vi "Plotsettings.vi"(4 "Decays 2":refnum<vi>, 5 "No of Channels":u32) -> ()   [LabVIEW 2009]
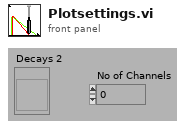
[diagram p1: front panel]
types:
  T1 = typedef "Settings.ctl" = cluster{"threshold":cluster{"max":u32, "min":u32}, "RGB or false color":bool, "16bit":bool, "log/lin axis":u16, "spotsize button":bool, "Pixelsize":u16, "autoscale x":bool, "autoscale y":bool, "correlation":bool, "ADC-Resolution":i32, "F2-lifetime":cluster{"display tau":bool, "display F2":bool, "Palette Number lifetime":enum32{"Gray", "Binary", "Gradient", "Rainbow", "Temperature"}, "Palette Number F2":enum32{"Gray", "Binary", "Gradient", "Rainbow", "Temperature"}, "max tau-Value":dbl, "min tau-Value":dbl, "max F2-Value":dbl, "min F2-Value":dbl}, "TAC-Window 1":u16, "TAC-Window 2":u16, "false color palette":cluster{"1":u32, "2":u32, "3":u32, "4":u32, "5":u32, "6":u32, "7":u32, "8":u32, "8 2":u32, "8 3":u32, "8 4":u32, "8 5":u32}, "rebinning":dbl}
  T2 = cluster{"1":u32, "2":u32, "3":u32, "4":u32, "5":u32, "6":u32, "7":u32, "8":u32, "8 2":u32, "8 3":u32, "8 4":u32, "8 5":u32}
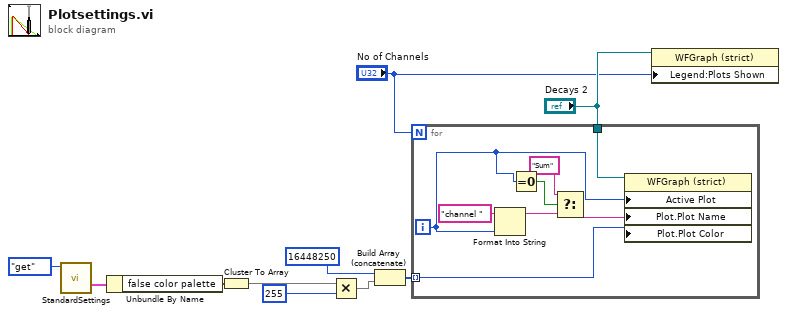
[diagram p0: block diagram]
diagram:
  n1 = call "StandardSettings.vi"("Enum"=enum16{"Load", "get", "Save", "set"}."get") -> ("StandardSettings"=w8:T1)  [unwired: 4 in]
  n2 = Unbundle By Name(w8) -> ("false color palette"=w7:T2)
  n3 = Cluster To Array(cluster=w7) -> (array=w3:u32[])
  n4 = Multiply(x=w3, y=255 ("Plot.Plot Color")) -> (x*y=w4:u32[])
  n5 = Build Array (concatenate)(u32 16448250 ("Plot.Plot Color"), w4) -> (w5:u32[])
  n6 = for {
    N: "No of Channels" -> [_]
    tunnel: "Decays 2" -> [w13]
    tunnel: w5 -> [w12] mode=indexing
    i -> [w11]
    n7 = Format Into String(initial string="channel ", w11) -> (resulting string=w16:string)  [unwired: 2 in, 1 out]
    n8 = Equal To 0?(x=w11) -> (x = 0?=w15:bool)
    n9 = Select(t="Sum", s=w15, f=w16) -> (s? t:f=w17:string)
    n10 = property on="Property Node" class="WFGraph (strict)"(reference=w13, "Active Plot"=w11, "Plot.Plot Name"=w17, "Plot.Plot Color"=w12) -> ()  [unwired: 1 in, 2 out]
  }
  n11 = property on="Property Node" class="WFGraph (strict)"(reference="Decays 2", "Legend:Plots Shown"="No of Channels") -> ()  [unwired: 1 in, 2 out]
